vi "8.8.2_글로벌.vi"() -> ()   [LabVIEW 2018]
panel:
  in  "while 정지":bool
  out "난수":dbl(graph)
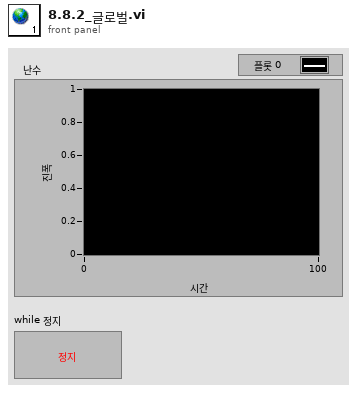
[diagram p1: front panel]
diagram:
